vi "Finish.vi"   [LabVIEW 2018]
doc: "This VI is called during exit. It can be used to close I/O refnums, save collected data, etc."
uses:
  <vilib>/Rock Robotics/WPI/Utilities/WPI_GetSetVariantRefNum.vi
types:
  T1 = typedef "WPI_CompressorDevRef.ctl" = cluster{"DevStatus":errorcluster, "Pneumatics Control Module":u8}
  T2 = typedef "WPI_SolenoidDevRef.ctl" = cluster{"DevStatus":errorcluster, "Pneumatics Control Module":u8, "Forward Solenoid Channel":T3, "Reverse Solenoid Channel":T3}
  T3 = typedef "WPI_SolenoidChannel.ctl" = enum8{"Solenoid 0", "Solenoid 1", "Solenoid 2", "Solenoid 3", "Solenoid 4", "Solenoid 5", "Solenoid 6", "Solenoid 7", "Invalid"}
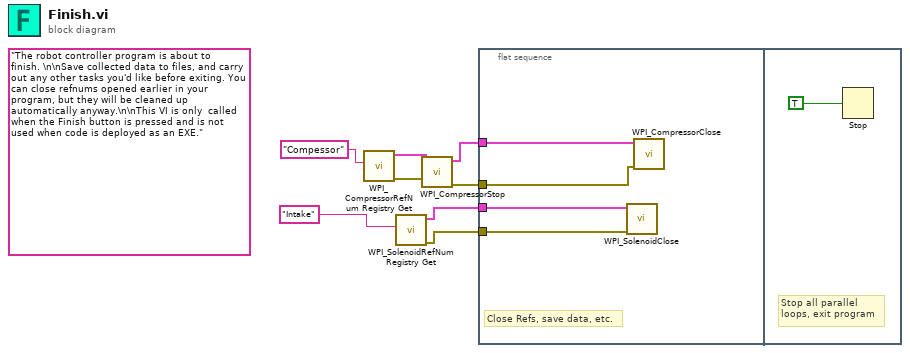
[diagram p0: block diagram]
diagram:
  (unwired) "The robot controller program is about to finish. \n\nSave collected data to files, and carry out any other tasks you'd like before exiting. You can close refnums opened earlier in your program, but they will be cleaned up automatically anyway.\n\nThis VI is only  called when the Finish button is pressed and is not used when code is deployed as an EXE."
  n1 = call <vilib>:"WPI_CompressorRefNum Registry Get.vi"("refnum name"="Compessor") -> ("error out"=w8:errorcluster, "CompressorDevRef"=w7:T1)  [unwired: 9 in]
  n2 = call <vilib>:"WPI_SolenoidRefNum Registry Get.vi"("refnum name"="Intake") -> ("error out"=w1:errorcluster, "SolenoidDevRef"=w2:T2)  [unwired: 9 in]
  n3 = call <vilib>:"WPI_CompressorStop.vi"("error in (no error)"=w8, "CompressorDevRef"=w7) -> ("error out"=w3:errorcluster, "CompressorDevRef"=w4:T1)  [unwired: 8 in]
  n4 = flat-sequence {
    tunnel: w4 -> [w12]
    tunnel: w3 -> [w11]
    tunnel: w2 -> [w10]
    tunnel: w1 -> [w9]
    frame #0 {
      # "Close Refs, save data, etc."
      n5 = call <vilib>:"WPI_SolenoidClose.vi"("error in (no error)"=w9, "SolenoidDevRef"=w10) -> ()  [unwired: 9 in, 1 out]
      n6 = call <vilib>:"WPI_CompressorClose.vi"("error in (no error)"=w11, "CompressorDevRef"=w12) -> ()  [unwired: 9 in, 1 out]
    }
    frame #1 {
      # "Stop all parallel\nloops, exit program"
      n7 = Stop(stop? (T)=TRUE ("Quit")) -> ()
    }
  }
